vi "celcius to fahrenheit.vi"() -> ()   [LabVIEW 2017]
panel:
  in  "stop":bool
  out "FAREN":dbl
  in  "Slide":dbl(slide) scale=0.0..50.0
  # "CELSIUS TO FAREINHEAT"
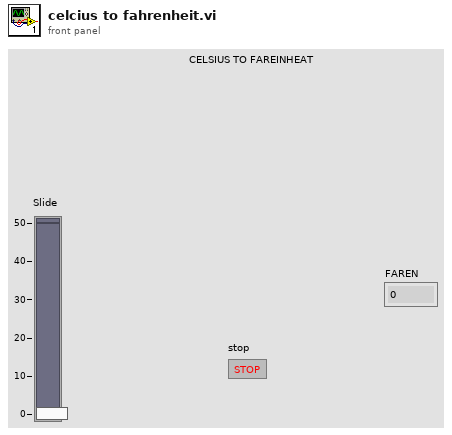
[diagram p1: front panel]
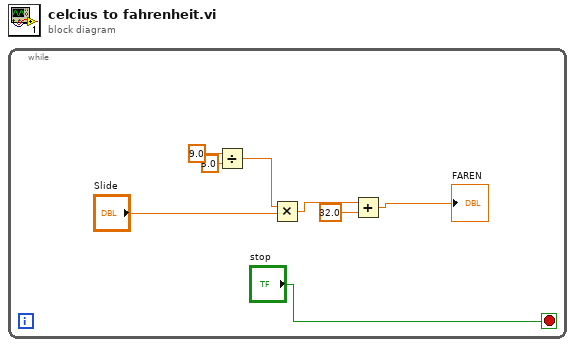
[diagram p0: block diagram]
diagram:
  n1 = while {
    stop <- "stop" stop-if-true
    n2 = Divide(x=9.0, y=5.0) -> (x/y=w6:dbl)
    n3 = Multiply(x=w6, y="Slide") -> (x*y=w5:dbl)
    n4 = Add(x=w5, y=32.0) -> (x+y=→"FAREN":dbl)
  }
